vi "CreateBarCode.vi"(8 "error in (no error)":errorcluster, 10 "Input":string, 11 "BarCode in":refnum<class "Linear Barcode.lvclass">) -> (0 "error out":errorcluster, 1 "Valid Value":bool, 2 "Barcode":picture, 3 "BarCode out":refnum<class "Linear Barcode.lvclass">)   [LabVIEW 2013, in "BarCodes.lvlib" / "Linear Barcode.lvclass"]
doc: "Creates a bar code to represent the specified text. If the text cannot be represented as a bar code in the format defined by this class, Valid Value will return false."
uses:
  Linear Barcode.lvclass
  BarCode/BarCode.lvclass
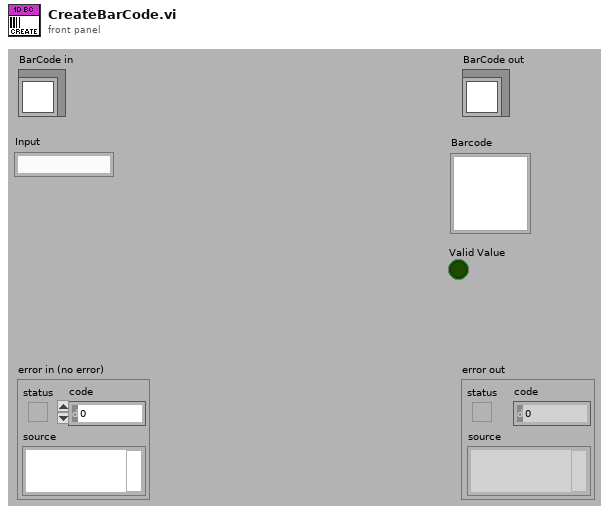
[diagram p1: front panel]
types:
  T1 = typedef "BarCodes.lvlib/BarCode.lvclass/Bar.ctl" = cluster{"Color":u32, "Width":u8}
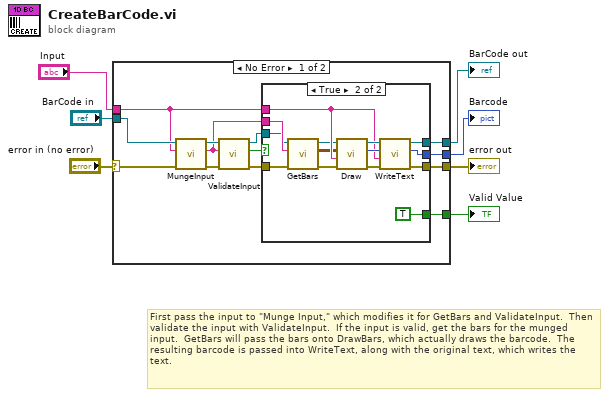
[diagram p0: block diagram]
diagram:
  # "First pass the input to \"Munge Input,\" which modifies it for GetBars and ValidateInput.  Then validate the input with ValidateInput.  If the input is valid, get the bars for the munged input.  GetBars will pass the bars onto DrawBars, which actually draws the barcode.  The resulting barcode is passed into WriteText, along with the original text, which writes the text."
  n1 = case shown="No Error" "error in (no error)" {
    selector: "error in (no error)" -> [w12 w39]
    tunnel: [w15 w39] -> w6
    tunnel: [w16 w38] -> w4
    tunnel: "BarCode in" -> [w13 w38]
    tunnel: [w18 _] -> w3
    tunnel: [w14 _] -> w2
    tunnel: "Input" -> [w8 _]
    frame No Error {
      n2 = call-dynamic "MungeInput.vi"("error in (no error)"=w12, "Input"=w8, "BarCode in"=w13) -> ("error out"=w11:errorcluster, "Munged Input"=w9:string, "BarCode out"=w10:refnum<class "Linear Barcode.lvclass">)  [unwired: 6 in]
      n3 = call-dynamic "ValidateInput.vi"("error in (no error)"=w11, "Input"=w9, "BarCode in"=w10) -> ("error out"=w19:errorcluster, "OK"=w20:bool, "BarCode out"=w17:refnum<class "Linear Barcode.lvclass">)  [unwired: 6 in]
      n4 = case shown="True" w20 {
        selector: w20 -> [w21 _]
        tunnel: w8 -> [_ w34]
        tunnel: w17 -> [w23 w25]
        tunnel: w19 -> [w22 w27]
        tunnel: [_ w32] -> w18
        tunnel: [w23 w31] -> w16
        tunnel: [w22 w33] -> w15
        tunnel: [w21 TRUE] -> w14
        tunnel: w9 -> [_ w26]
        frame False {
        }
        frame True {
          n5 = call-dynamic "GetBars.vi"("error in (no error)"=w27, "Munged Input"=w26, "BarCode in"=w25) -> ("error out"=w29:errorcluster, "BarWidths"=w24:T1[][], "BarCode out"=w28:refnum<class "Linear Barcode.lvclass">)  [unwired: 6 in]
          n6 = call "Draw.vi"("error in (no error)"=w29, "Text"=w34, "Bars"=w24, "2D Barcode in"=w28) -> ("error out"=w37:errorcluster, "new picture"=w36:picture, "2D Barcode out"=w35:refnum<class "Linear Barcode.lvclass">)  [unwired: 5 in]
          n7 = call "WriteText.vi"("error in (no error)"=w37, "Original Input"=w34, "Picture In"=w36, "BarCode in"=w35) -> ("error out"=w33:errorcluster, "Picture Out"=w32:picture, "BarCode out"=w31:refnum<class "Linear Barcode.lvclass">)  [unwired: 5 in]
        }
      }
    }
    frame Error {
    }
  }
  "error out" <- w6
  "BarCode out" <- w4
  "Barcode" <- w3
  "Valid Value" <- w2
